vi "Quench.vi"() -> ()   [LabVIEW 2013]
uses:
  <vilib>/NI/Current Value Table/Read tags into grouped data.vi
  <vilib>/NI/Current Value Table/Read Index Set.vi
  <vilib>/NI/Current Value Table/DataTypes/Double_Read Index Set.vi
  <vilib>/NI/Current Value Table/DataTypes/Array of String_Read Index Set.vi
  <vilib>/NI/Current Value Table/DataTypes/Array of Boolean_Read Index Set.vi
  <vilib>/NI/Current Value Table/DataTypes/Array of Single_Read Index Set.vi
  <vilib>/NI/Current Value Table/DataTypes/Array of Double_Read Index Set.vi
  <vilib>/NI/Current Value Table/DataTypes/Array of I8_Read Index Set.vi
  <vilib>/NI/Current Value Table/DataTypes/Array of I16_Read Index Set.vi
  <vilib>/NI/Current Value Table/DataTypes/Array of I32_Read Index Set.vi
  <vilib>/NI/Current Value Table/DataTypes/Array of I64_Read Index Set.vi
  <vilib>/NI/Current Value Table/DataTypes/Array of U64_Read Index Set.vi
  <vilib>/NI/Current Value Table/DataTypes/Array of U32_Read Index Set.vi
  <vilib>/NI/Current Value Table/DataTypes/Array of U16_Read Index Set.vi
  <vilib>/NI/Current Value Table/DataTypes/Array of U8_Read Index Set.vi
  <vilib>/NI/Current Value Table/DataTypes/Boolean_Read Index Set.vi
  <vilib>/NI/Current Value Table/DataTypes/String_Read Index Set.vi
  <vilib>/NI/Current Value Table/DataTypes/U8_Read Index Set.vi
  <vilib>/NI/Current Value Table/DataTypes/U16_Read Index Set.vi
  <vilib>/NI/Current Value Table/DataTypes/U32_Read Index Set.vi
  <vilib>/NI/Current Value Table/DataTypes/U64_Read Index Set.vi
  <vilib>/NI/Current Value Table/DataTypes/I8_Read Index Set.vi
  <vilib>/NI/Current Value Table/DataTypes/I16_Read Index Set.vi
  <vilib>/NI/Current Value Table/DataTypes/I32_Read Index Set.vi
  <vilib>/NI/Current Value Table/DataTypes/I64_Read Index Set.vi
  <vilib>/NI/Current Value Table/DataTypes/Single_Read Index Set.vi
  <vilib>/NI/Current Value Table/FGVs/Group Memory.vi
  <vilib>/NI/Current Value Table/Memory Block.vi
  <vilib>/NI/Current Value Table/DataTypes/Double_Memory Block.vi
  <vilib>/NI/Current Value Table/DataTypes/Array of String_Memory Block.vi
  <vilib>/NI/Current Value Table/DataTypes/Array of Boolean_Memory Block.vi
  <vilib>/NI/Current Value Table/DataTypes/Array of Single_Memory Block.vi
  <vilib>/NI/Current Value Table/DataTypes/Array of Double_Memory Block.vi
  <vilib>/NI/Current Value Table/DataTypes/Array of I8_Memory Block.vi
  <vilib>/NI/Current Value Table/DataTypes/Array of I16_Memory Block.vi
  <vilib>/NI/Current Value Table/DataTypes/Array of I32_Memory Block.vi
  <vilib>/NI/Current Value Table/DataTypes/Array of I64_Memory Block.vi
  <vilib>/NI/Current Value Table/DataTypes/Array of U64_Memory Block.vi
  <vilib>/NI/Current Value Table/DataTypes/Array of U32_Memory Block.vi
  <vilib>/NI/Current Value Table/DataTypes/Array of U16_Memory Block.vi
  <vilib>/NI/Current Value Table/DataTypes/Array of U8_Memory Block.vi
  <vilib>/NI/Current Value Table/DataTypes/Boolean_Memory Block.vi
  <vilib>/NI/Current Value Table/DataTypes/String_Memory Block.vi
  <vilib>/NI/Current Value Table/DataTypes/U8_Memory Block.vi
  <vilib>/NI/Current Value Table/DataTypes/U16_Memory Block.vi
  <vilib>/NI/Current Value Table/DataTypes/U32_Memory Block.vi
  <vilib>/NI/Current Value Table/DataTypes/U64_Memory Block.vi
  <vilib>/NI/Current Value Table/DataTypes/I8_Memory Block.vi
  <vilib>/NI/Current Value Table/DataTypes/I16_Memory Block.vi
  <vilib>/NI/Current Value Table/DataTypes/I32_Memory Block.vi
  <vilib>/NI/Current Value Table/DataTypes/I64_Memory Block.vi
  <vilib>/NI/Current Value Table/DataTypes/Single_Memory Block.vi
  <vilib>/NI/Current Value Table/Current Value Table.lvlib
panel:
  out "error out":errorcluster
  in  "Boolean":bool
  out "PI-421":dbl format="%.1f"
  out "PI-411":dbl format="%.1f"
  in  "FT-410":dbl
  in  "FT-420":dbl
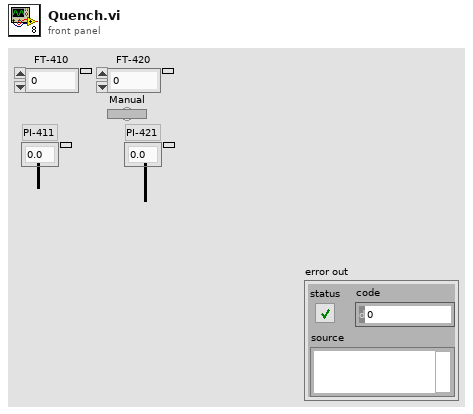
[diagram p1: front panel]
types:
  T1 = typedef "Current Value Table.lvlib/Group Data.ctl" = cluster{"Double":dbl[], "Single":sgl[], "I64":i64[], "I32":i32[], "I16":i16[], "I8":i8[], "U64":u64[], "U32":u32[], "U16":u16[], "U8":u8[], "String":string[], "Boolean":bool[], "Array of U8":cluster{"U8 Array":u8[]}[], "Array of U16":cluster{"U16 Array":u16[]}[], "Array of U32":cluster{"U32 Array":u32[]}[], "Array of U64":cluster{"U64 Array":u64[]}[], "Array of I64":cluster{"I64 Array":i64[]}[], "Array of I32":cluster{"I32 Array":i32[]}[], "Array of I16":cluster{"I16 Array":i16[]}[], "Array of I8":cluster{"I8 Array":i8[]}[], "Array of Double":cluster{"DBL Array":dbl[]}[], "Array of Single":cluster{"SGL Array":sgl[]}[], "Array of Boolean":cluster{"Boolean Array":bool[]}[], "Array of String":cluster{"String Array":string[]}[]}
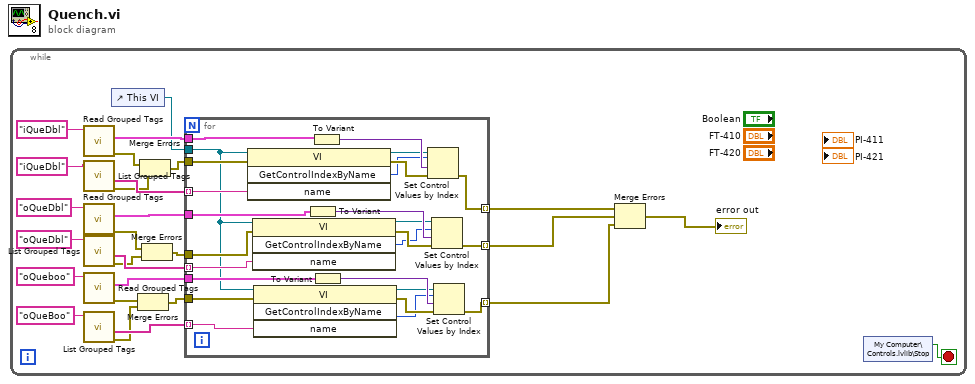
[diagram p0: block diagram]
diagram:
  n1 = while {
    stop <- w1 stop-if-true
    n2 = call <vilib>:"Read Grouped Tags.vi"("Group"="iQueDbl") -> ("error out"=w23:errorcluster, "Data"=w26:T1)  [unwired: 9 in]
    n3 = call <vilib>:"List Grouped Tags.vi"("Group"="iQueDbl") -> ("error out"=w22:errorcluster, "Tags Out"=w27:string[])  [unwired: 9 in]
    n4 = call <vilib>:"Read Grouped Tags.vi"("Group"="oQueDbl") -> ("error out"=w17:errorcluster, "Data"=w18:T1)  [unwired: 9 in]
    n5 = call <vilib>:"List Grouped Tags.vi"("Group"="oQueDbl") -> ("error out"=w16:errorcluster, "Tags Out"=w19:string[])  [unwired: 9 in]
    n6 = call <vilib>:"Read Grouped Tags.vi"("Group"="oQueboo") -> ("error out"=w10:errorcluster, "Data"=w11:T1)  [unwired: 9 in]
    n7 = call <vilib>:"List Grouped Tags.vi"("Group"="oQueBoo") -> ("error out"=w9:errorcluster, "Tags Out"=w12:string[])  [unwired: 9 in]
    n8 = control-ref of="This VI"() -> (w20:refnum<vi>)
    n9 = Merge Errors(w10, w9) -> (w8:errorcluster)
    n10 = Merge Errors(w23, w22) -> (w21:errorcluster)
    n11 = Merge Errors(w17, w16) -> (w15:errorcluster)
    n12 = for {
      tunnel: w27 -> [w50] mode=indexing
      tunnel: w26 -> [w49]
      tunnel: w21 -> [w48]
      tunnel: w20 -> [w32]
      tunnel: w19 -> [w41] mode=indexing
      tunnel: w18 -> [w40]
      tunnel: w15 -> [w39]
      tunnel: w12 -> [w34] mode=indexing
      tunnel: w11 -> [w33]
      tunnel: w8 -> [w31]
      tunnel: [w30] -> w7 mode=indexing
      tunnel: [w29] -> w6 mode=indexing
      tunnel: [w28] -> w5 mode=indexing
      n13 = invoke class="VI" method="GetControlIndexByName"(reference=w32, error in=w48, "name"=w50) -> (reference out=w47:refnum<vi>, error out=w52:errorcluster, "GetControlIndexByName"=w46:i32)  [unwired: 1 in, 1 out]
      n14 = invoke class="VI" method="GetControlIndexByName"(reference=w32, error in=w39, "name"=w41) -> (reference out=w43:refnum<vi>, error out=w45:errorcluster, "GetControlIndexByName"=w42:i32)  [unwired: 1 in, 1 out]
      n15 = invoke class="VI" method="GetControlIndexByName"(reference=w32, error in=w31, "name"=w34) -> (reference out=w36:refnum<vi>, error out=w38:errorcluster, "GetControlIndexByName"=w35:i32)  [unwired: 1 in, 1 out]
      n16 = To Variant(anything=w40) -> (Variant=w44:variant)
      n17 = To Variant(anything=w49) -> (Variant=w51:variant)
      n18 = To Variant(anything=w33) -> (Variant=w37:variant)
      n19 = Set Control Values by Index(0:w47, 1:w46, 2:w51, 3:w52) -> (11:w30:errorcluster)
      n20 = Set Control Values by Index(0:w43, 1:w42, 2:w44, 3:w45) -> (11:w29:errorcluster)
      n21 = Set Control Values by Index(0:w36, 1:w35, 2:w37, 3:w38) -> (11:w28:errorcluster)
    }
    n22 = Merge Errors(w7, w6, w5) -> (→"error out":errorcluster)
    n23 = shared-variable "My Computer\\Controls.lvlib\\Stop"() -> (w1:bool)  [unwired: 1 in, 1 out]
  }
